vi "Add Scan Engine Custom Device.vi"(8 "error in":errorcluster, 10 "settings":T1={"sync to scan"=FALSE, "scan engine decimation"=1, "delay after FPGA load (s)"=1}, 11 "target in":refnum<k39>) -> (0 "error out":errorcluster, 2 "scan engine custom device ref":T2 format="%.0x", 3 "target out":refnum<k39>)   [LabVIEW 2020, in "Scan Engine Scripting.lvlib"]
doc: "Adds the Scan Engine and EtherCAT custom device to the selected target."
uses:
  Scan Engine Scripting.lvlib
  C:/Users/Administrator/Desktop/Jatin/All DNC DLLs/NationalInstruments.VeriStand.SystemDefinitionAPI.dll
  Jatin/All DNC DLLs/NationalInstruments.VeriStand.SystemDefinitionAPI.dll
  Shared/Globals/Scan Engine GUIDs.vi
  Shared/SEECD Shared.lvlib
  System Explorer/SEECD System Explorer.lvlib
  Shared/Globals/Error Strings.vi
  Utility/Ref Constants.vi
  <vilib>/NI VeriStand/Custom Device API/Custom Device Item Ref.ctl
  <vilib>/NI VeriStand/Custom Device API/Custom Device API.lvlib
  Shared/Type Defs/Main Settings.ctl
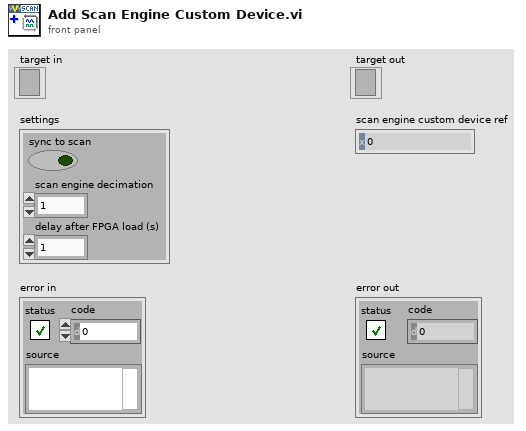
[diagram p1: front panel]
types:
  T1 = typedef "SEECD Shared.lvlib/Main Settings.ctl" = cluster{"sync to scan":bool, "scan engine decimation":u16, "delay after FPGA load (s)":u16}
  T2 = typedef "Custom Device API.lvlib/Custom Device Item Ref.ctl" = u64
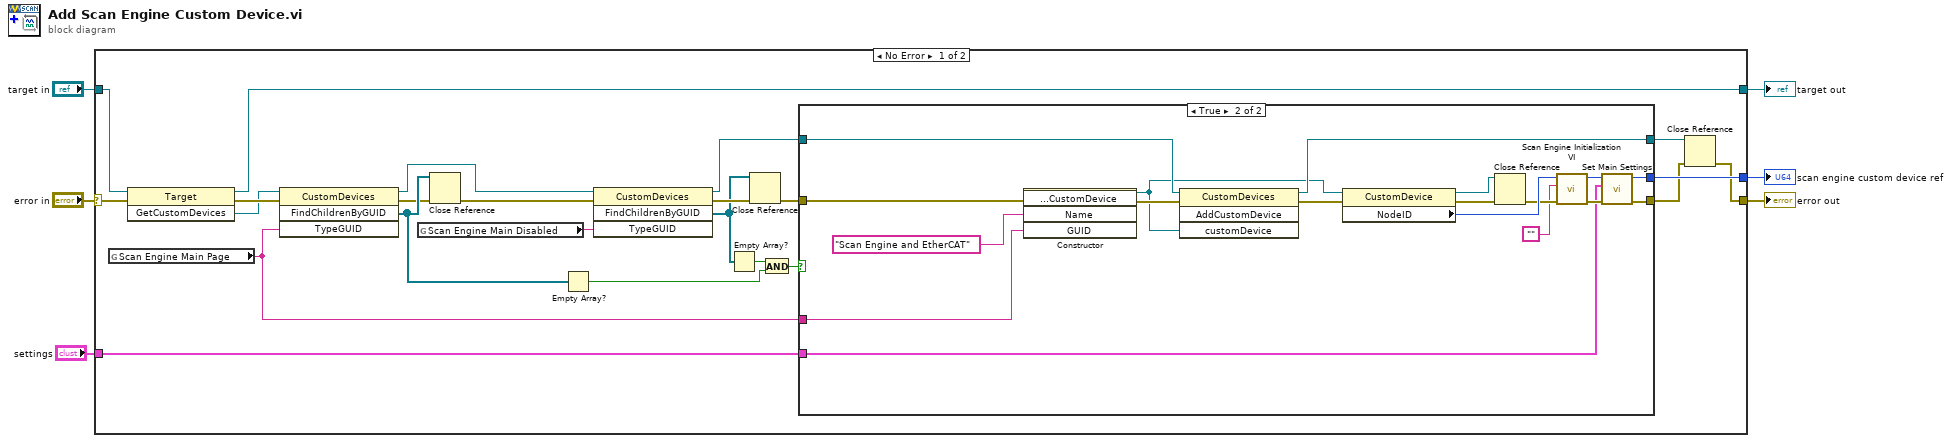
[diagram p0: block diagram]
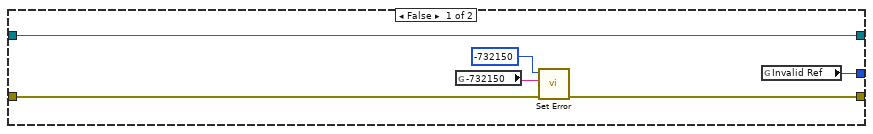
[diagram p2: hidden frame]
diagram:
  n1 = case shown="No Error" "error in" {
    selector: "error in" -> [w19 w55]
    tunnel: [w22 w55] -> w6
    tunnel: "target in" -> [w20 w54]
    tunnel: [w29 w54] -> w3
    tunnel: [w28 _] -> w2
    tunnel: "settings" -> [w17 _]
    frame No Error {
      n2 = global read "Scan Engine GUIDs.vi" "Scan Engine Main Page"() -> (w18:string)
      n3 = invoke class="Target" method="GetCustomDevices"(reference=w20, error in=w19) -> (reference out=w29:refnum<k39>, error out=w27:errorcluster, "GetCustomDevices"=w21:refnum<k39>)  [unwired: 1 in]
      n4 = invoke class="CustomDevices" method="FindChildrenByGUID"(reference=w21, error in=w27, "TypeGUID"=w18) -> (reference out=w13:refnum<k39>, error out=w25:errorcluster, "FindChildrenByGUID"=w26:refnum<k39>[])  [unwired: 1 in, 1 out]
      n5 = global read "Scan Engine GUIDs.vi" "Scan Engine Main Disabled"() -> (w15:string)
      n6 = Close Reference(reference=w26, error in (no error)=w25) -> (error out=w16:errorcluster)
      n7 = Empty Array?(array=w26) -> (empty?=w9:bool)
      n8 = invoke class="CustomDevices" method="FindChildrenByGUID"(reference=w13, error in=w16, "TypeGUID"=w15) -> (reference out=w7:refnum<k39>, error out=w14:errorcluster, "FindChildrenByGUID"=w11:refnum<k39>[])  [unwired: 1 in, 1 out]
      n9 = Empty Array?(array=w11) -> (empty?=w10:bool)
      n10 = Close Reference(reference=w11, error in (no error)=w14) -> (error out=w12:errorcluster)
      n11 = And(x=w10, y=w9) -> (x .and. y?=w8:bool)
      n12 = case shown="True" w8 {
        tunnel: [w31 w37] -> w23
        tunnel: [w30 w39] -> w28
        tunnel: w7 -> [w35 w49]
        tunnel: w12 -> [w32 w47]
        tunnel: [w35 w48] -> w24
        tunnel: w18 -> [_ w45]
        tunnel: w17 -> [_ w36]
        frame False {
          n13 = global read "Error Strings.vi" "-732150"() -> (w33:string)
          n14 = call "Set Error.vi"("error in (no error)"=w32, "Message"=w33, "Code"=-732150 ("error code (0)")) -> ("error out"=w31:errorcluster)  [unwired: 8 in]
          n15 = global read "Ref Constants.vi" "Invalid Ref"() -> (w30:T2)
        }
        frame True {
          n16 = constructor class="CustomDevice"(error in=w47, "Name"="Scan Engine and EtherCAT", "GUID"=w45) -> (reference out=w46:refnum<k39>, error out=w53:errorcluster)  [unwired: 2 in, 3 out]
          n17 = invoke class="CustomDevices" method="AddCustomDevice"(reference=w49, error in=w53, "customDevice"=w46) -> (reference out=w48:refnum<k39>, error out=w52:errorcluster)  [unwired: 1 in, 2 out]
          n18 = property class="CustomDevice"(reference=w46, error in=w52) -> (reference out=w51:refnum<k39>, error out=w50:errorcluster, "NodeID"=w44:u64)
          n19 = Close Reference(reference=w51, error in (no error)=w50) -> (error out=w43:errorcluster)
          n20 = call "Scan Engine Initialization VI.vi"("error in (no error)"=w43, "Custom XML"="", "Device Item Ref in"=w44) -> ("error out"=w38:errorcluster, "Device Item Ref out"=w40:T2)  [unwired: 7 in]
          n21 = call "Set Main Settings.vi"("error in"=w38, "settings"=w36, "scan engine custom device ref in"=w40) -> ("error out"=w37:errorcluster, "scan engine custom device ref out"=w39:T2)  [unwired: 7 in]
        }
      }
      n22 = Close Reference(reference=w24, error in (no error)=w23) -> (error out=w22:errorcluster)
    }
    frame Error {
    }
  }
  "target out" <- w3
  "error out" <- w6
  "scan engine custom device ref" <- w2
